vi "GEA2 Serial Get STX.vi"(8 "Error In":errorcluster, 9 "ReadArray":u8[](array[numeric]), 10 "Current Read Index in":i32, 11 "Total Bytes Read":i32) -> (0 "Error Out":errorcluster, 1 "Complete Message":bool, 2 "Current Read Index out":i32, 3 "Read Array Out":u8[](array[numeric]))   [LabVIEW 2014]
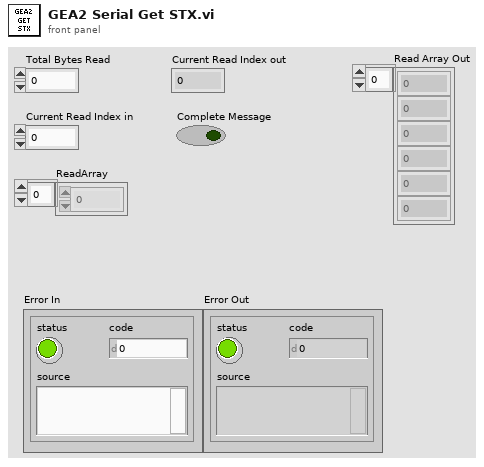
[diagram p1: front panel]
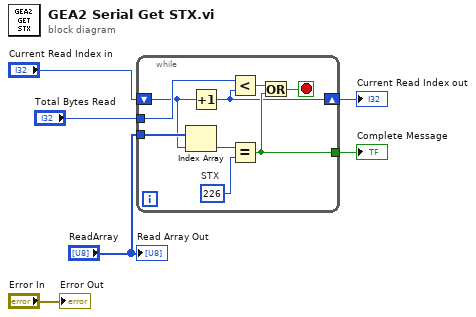
[diagram p0: block diagram]
diagram:
  n1 = while {
    tunnel: [w12] -> w2
    tunnel: "Total Bytes Read" -> [w11]
    shift-right: [w8] -> w6
    shift-left: "Current Read Index in" -> [w9]
    tunnel: "ReadArray" -> [w15]
    stop <- w13 stop-if-true
    w7 = u8 226  # STX
    n2 = Index Array(array=w15, index=w9) -> (element=w14:u8)
    n3 = Increment(x=w9) -> (x+1=w8:i32)
    n4 = Less?(x=w11, y=w8) -> (x < y?=w10:bool)
    n5 = Equal?(x=w14, y=w7) -> (x = y?=w12:bool)
    n6 = Or(x=w10, y=w12) -> (x .or. y?=w13:bool)
  }
  "Current Read Index out" <- w6
  "Complete Message" <- w2
  "Error Out" <- "Error In"
  "Read Array Out" <- "ReadArray"
